vi "1553 Channels to Address Based Handles.vi"(8 "error in":errorcluster, 11 "custom device ref":T4 format="%.0x") -> (0 "error out":errorcluster, 1 "address based channel handles":T1 {"acyclic frame trigger handles"."handle" format="%.0x"; "start stop handles"."stop handle" format="%.0x"; "start stop handles"."start handle" format="%.0x"}, 2 "address based channels":T4[](array[typedef]) format="%.0x", 3 "custom device ref out":T4 format="%.0x")   [LabVIEW 2020, in "AIM MIL-STD-1553 Engine.lvlib" / "Implementation.lvlib" / "Address Based Execution Unit.lvclass"]
uses:
  Address Based Execution Unit.lvclass
  <vilib>/NI VeriStand/Custom Device API/Custom Device Item Ref.ctl
  <vilib>/NI VeriStand/Custom Device API/Custom Device API.lvlib
  Scripting/AIM MIL-STD-1553 Scripting.lvlib
  Shared/Address.ctl
  Start Stop Channel Handles.ctl
  1553 Address Based Handles.ctl
  Acyclic Frame Trigger Handle.ctl
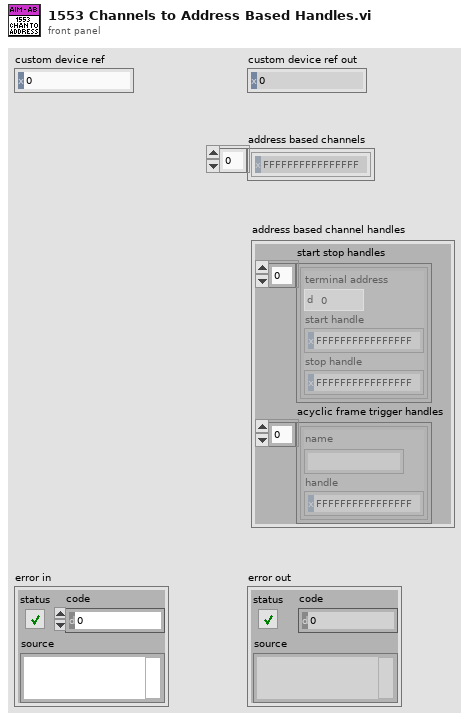
[diagram p1: front panel]
types:
  T1 = typedef "AIM MIL-STD-1553 Engine.lvlib/Implementation.lvlib/Address Based Execution Unit.lvclass/1553 Address Based Handles.ctl" = cluster{"start stop handles":T2[], "acyclic frame trigger handles":T5[]}
  T2 = typedef "AIM MIL-STD-1553 Engine.lvlib/Implementation.lvlib/Address Based Execution Unit.lvclass/Start Stop Channel Handles.ctl" = cluster{"terminal address":T3, "start handle":T4, "stop handle":T4}
  T3 = typedef "Address.ctl" = u16
  T4 = typedef "Custom Device API.lvlib/Custom Device Item Ref.ctl" = u64
  T5 = typedef "AIM MIL-STD-1553 Engine.lvlib/Implementation.lvlib/Address Based Execution Unit.lvclass/Acyclic Frame Trigger Handle.ctl" = cluster{"name":string, "handle":T4}
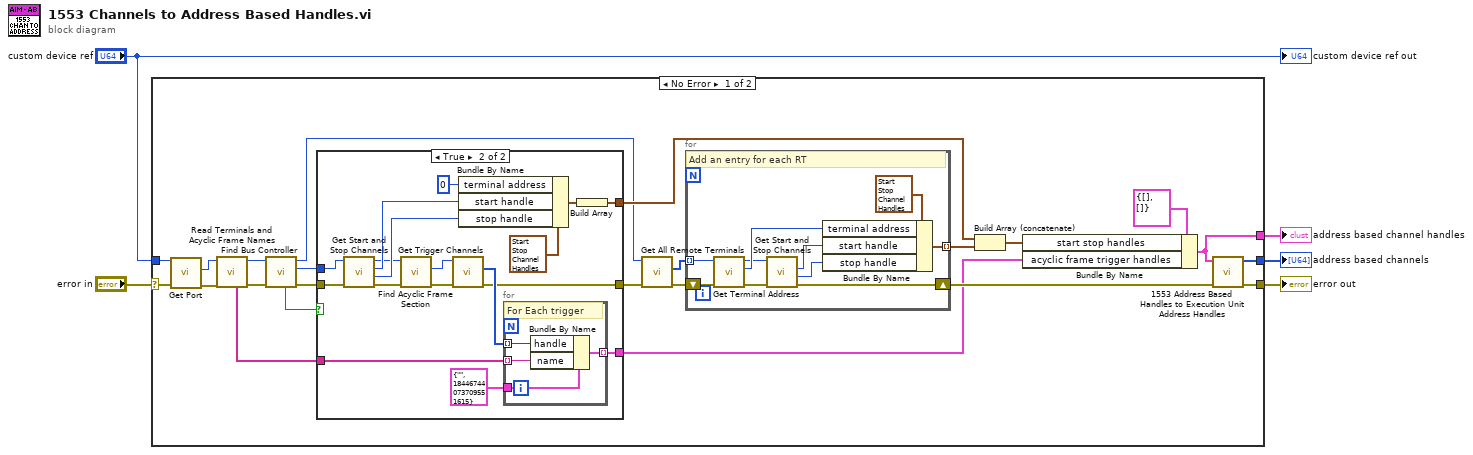
[diagram p0: block diagram]
diagram:
  n1 = case shown="No Error" "error in" {
    selector: "error in" -> [w7 w61]
    tunnel: "custom device ref" -> [w6 _]
    tunnel: [w27 w61] -> w4
    tunnel: [w26 _] -> w3
    tunnel: [w25 _] -> w1
    frame No Error {
      n2 = call "Get Port.vi"("error in"=w7, "custom device ref"=w6) -> ("error out"=w8:errorcluster, "port"=w9:T4)  [unwired: 6 in, 2 out]
      n3 = call "Read Terminals and Acyclic Frame Names.vi"("error in"=w8, "port"=w9) -> ("error out"=w14:errorcluster, "port out"=w15:T4, "acyclic frame names"=w16:string[])  [unwired: 5 in, 2 out]
      n4 = call "Find Bus Controller.vi"("error in"=w14, "port"=w15) -> ("error out"=w22:errorcluster, "bus controller"=w18:T4, "port out"=w10:T4, "found?"=w11:bool)  [unwired: 6 in]
      n5 = case shown="True" w11 {
        tunnel: w22 -> [w29 w46]
        tunnel: w18 -> [_ w40]
        tunnel: [_ w37] -> w17
        tunnel: w16 -> [_ w36]
        tunnel: [_ w32] -> w13
        tunnel: [w29 w33] -> w12
        frame False {
        }
        frame True {
          n6 = call "Get Start and Stop Channels.vi"("error in"=w46, "terminal in"=w40) -> ("error out"=w35:errorcluster, "stop channel"=w43:T4, "start channel"=w44:T4, "terminal out"=w34:T4)  [unwired: 5 in, 1 out]
          n7 = call "Find Acyclic Frame Section.vi"("error in"=w35, "bus controller in"=w34) -> ("error out"=w39:errorcluster, "acyclic frames section"=w41:T4)  [unwired: 6 in, 2 out]
          n8 = call "Get Trigger Channels.vi"("error in"=w39, "acyclic frames section in"=w41) -> ("error out"=w33:errorcluster, "acyclic frame triggers"=w38:T4[])  [unwired: 6 in, 2 out]
          n9 = Bundle By Name(cluster=T2 {"terminal address"=0, "start handle"=18446744073709551615, "stop handle"=18446744073709551615} ("start stop handle"), "terminal address"=T3 0, "start handle"=w44, "stop handle"=w43) -> (w31:T2)
          n10 = for {
            tunnel: w36 -> [w48] mode=indexing
            tunnel: w38 -> [w50] mode=indexing
            tunnel: [w49] -> w37 mode=indexing
            tunnel: T5 {"name"="", "handle"=18446744073709551615} ("acyclic frame trigger handle") -> [w47]
            # "For Each trigger"
            n11 = Bundle By Name(cluster=w47, "handle"=w50, "name"=w48) -> (w49:T5)
          }
          n12 = Build Array(w31) -> (w32:T2[])
        }
      }
      n13 = call "Get All Remote Terminals.vi"("error in"=w12, "port in"=w10) -> ("error out"=w24:errorcluster, "remote terminals"=w23:T4[])  [unwired: 7 in, 1 out]
      n14 = for {
        shift-right: [w52] -> w28
        shift-left: w24 -> [w59]
        tunnel: w23 -> [w58] mode=indexing
        tunnel: [w51] -> w21 mode=indexing
        # "Add an entry for each RT"
        n15 = call "Get Terminal Address.vi"("error in"=w59, "remote terminal in"=w58) -> ("error out"=w56:errorcluster, "terminal address"=w57:T3, "remote terminal out"=w55:T4)  [unwired: 6 in, 1 out]
        n16 = call "Get Start and Stop Channels.vi"("error in"=w56, "terminal in"=w55) -> ("error out"=w52:errorcluster, "stop channel"=w53:T4, "start channel"=w54:T4)  [unwired: 5 in, 2 out]
        n17 = Bundle By Name(cluster=T2 {"terminal address"=0, "start handle"=18446744073709551615, "stop handle"=18446744073709551615} ("start stop handle"), "terminal address"=w57, "start handle"=w54, "stop handle"=w53) -> (w51:T2)
      }
      n18 = Build Array (concatenate)(w13, w21) -> (w19:T2[])
      n19 = Bundle By Name(cluster=T1 {"start stop handles"=[], "acyclic frame trigger handles"=[]} ("1553 start stop handles"), "start stop handles"=w19, "acyclic frame trigger handles"=w17) -> (w25:T1)
      n20 = call "1553 Address Based Handles to Execution Unit Address Handles.vi"("error in"=w28, "1553 address based channel handles"=w25) -> ("error out"=w27:errorcluster, "address based channels"=w26:T4[])  [unwired: 8 in]
    }
    frame Error {
    }
  }
  "error out" <- w4
  "address based channels" <- w3
  "address based channel handles" <- w1
  "custom device ref out" <- "custom device ref"
